vi "Keyence U8 array to I32.vi"(11 "U8 Array":u8[](array[numeric])) -> (3 "I32":i32)   [LabVIEW 2018]
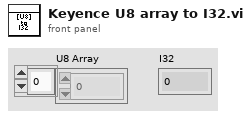
[diagram p1: front panel]
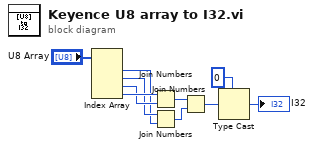
[diagram p0: block diagram]
diagram:
  n1 = Index Array(array="U8 Array") -> (element #1=w4:u8, element #2=w5:u8, element #3=w6:u8, element #4=w7:u8)  [unwired: 4 in]
  n2 = Join Numbers(hi=w7, lo=w6) -> ((hi.lo)=w8:u16)
  n3 = Join Numbers(hi=w5, lo=w4) -> ((hi.lo)=w9:u16)
  n4 = Join Numbers(hi=w8, lo=w9) -> ((hi.lo)=w2:u32)
  n5 = Type Cast(type=0 ("(hi.lo)"), x=w2) -> (*(type *) &x=→"I32":i32)
